vi "AB_CanEmbedTypeLibrary.vi"(8 "error in (no error)":errorcluster) -> (0 "error out":errorcluster, 3 "Can embed type library?":bool)   [LabVIEW 2020]
panel:
  in  "LabVIEW_DB.Application":refnum<k7>
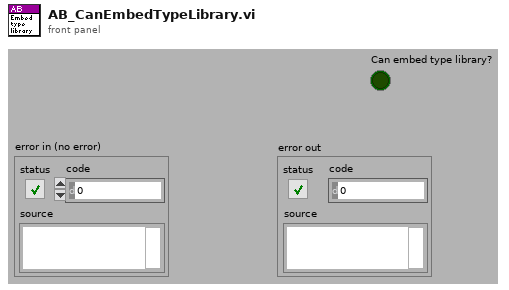
[diagram p1: front panel]
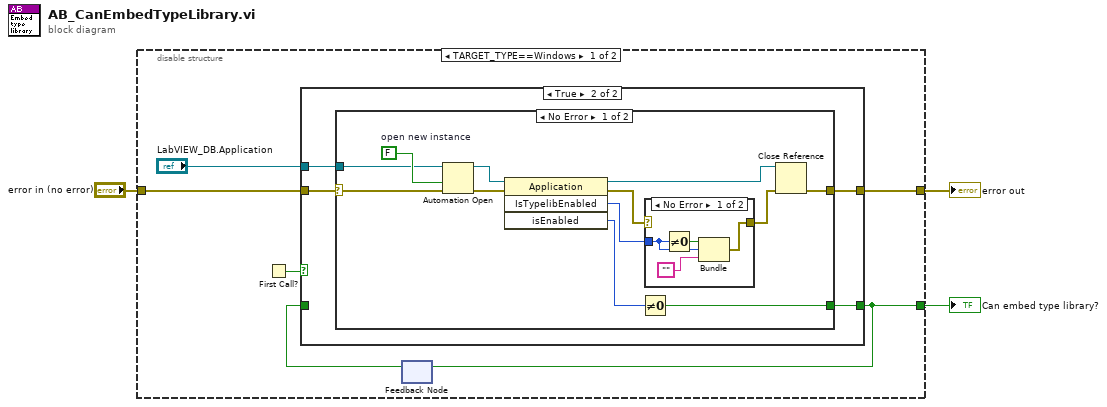
[diagram p0: block diagram]
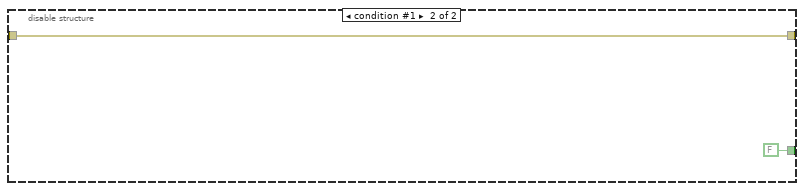
[diagram p5: hidden frame]
diagram:
  n1 = disable-structure shown="TARGET_TYPE==Windows" {
    disable-tunnel: [w9 FALSE] -> w3
    disable-tunnel: [w6 w35] -> w2
    disable-tunnel: "error in (no error)" -> [w4 w35]
    frame condition #0 (active) {
      n2 = First Call?() -> (First Call?: T/F=w7:bool)
      n3 = feedback #1() -> (w8:bool)  [unwired: 1 in]
      n4 = case shown="True" w7 {
        tunnel: [w11 w15] -> w9
        tunnel: w8 -> [w11 _]
        tunnel: [w10 w14] -> w6
        tunnel: "LabVIEW_DB.Application" -> [_ w13]
        tunnel: w4 -> [w10 w12]
        frame False {
        }
        frame True {
          n5 = case shown="No Error" w12 {
            selector: w12 -> [w16 w33]
            tunnel: [w19 _] -> w15
            tunnel: [w18 w33] -> w14
            tunnel: w13 -> [w17 _]
            frame No Error {
              w27 = FALSE  # open new instance
              n6 = Automation Open(error in (no error)=w16, Automation Refnum=w17, 9:w27) -> (Automation Refnum=w25:refnum<k7>, error out=w23:errorcluster)  [unwired: 1 out]
              n7 = invoke class="Application" method="IsTypelibEnabled"(reference=w25, error in=w23) -> (reference out=w24:refnum<k7>, error out=w21:errorcluster, "IsTypelibEnabled"=w22:i32, "isEnabled"=w26:i32)  [unwired: 2 in]
              n8 = Not Equal To 0?(x=w26) -> (x != 0?=w19:bool)
              n9 = case shown="No Error" w21 {
                selector: w21 -> [_ w32]
                tunnel: w22 -> [w30 _]
                tunnel: [w29 w32] -> w20
                frame No Error {
                  n10 = Not Equal To 0?(x=w30) -> (x != 0?=w31:bool)
                  n11 = Bundle(w31, "IsTypelibEnabled"=w30, "") -> (w29:cluster{bool, "IsTypelibEnabled":i32, string})  [unwired: 1 out]
                }
                frame Error {
                }
              }
              n12 = Close Reference(reference=w24, error in (no error)=w20) -> (error out=w18:errorcluster)
            }
            frame Error {
            }
          }
        }
      }
      n13 = feedback-in #1(w9) -> ()
    }
    frame condition #1 {
    }
  }
  "Can embed type library?" <- w3
  "error out" <- w2
